vi "FPGA Main Default.vi"() -> ()   [LabVIEW 2021]
doc: "The myRIO v1.1 FPGA Shipping Personality. This personality contains support for:\n- 2 Analog Input Interrupt channel\n- 4 Digital Input Interrupt channel\n- 1 Timer\n- 1 Accelerometer\n- 1 Button\n- 4 LED\n- 10 Analog Input channels with 1 Sample\n- 6 Analog Output channels with 1 Sample\n- 40 Digital I/O channels with 1 Sample\n- 2 I2C channels\n- 4 Encoder channels\n- 6 PWM channels\n- 2 SPI channels"
uses:
  Sub VIs/Utilities/Start Boolean.ctl
  <vilib>/Platform/TimedLoop/XDataNode/timing_clust.ctl
  <vilib>/Platform/TimedLoop/XDataNode/nitl_modes.ctl
  <vilib>/Platform/TimedLoop/XDataNode/wakeup.ctl
  <vilib>/rvi/Emulation/niFpgaGetClockAttributes.vi
  <vilib>/rvi/Emulation/niFpgaSctlEmulationGetInTimedLoop.vi
  <vilib>/rvi/Emulation/niFpgaEmulationReportErrorSimple.vi
  <vilib>/rvi/eio/common/nirviEmuTemplateMethod_errors.vi
  <vilib>/rvi/Emulation/niFpgaCriticalErrorInLSC.vi
  <vilib>/rvi/Emulation/niFpgaProcessEmulError.vi
  <vilib>/rvi/Emulation/niFpgaEmulationIsFPGAContextNoSignature.vi
  <vilib>/rvi/errors/niFpgaSetErrorForExecOnDevCompSimple.vi
  <vilib>/rvi/eio/common/nirviEmuReportErrorAndStop.vi
  <vilib>/rvi/DataTransferAndStorage/Container/Common/niFpgaContainerGetUniqueNameForEmu.vi
  <vilib>/rvi/FIFO/Fifo_Resource/nirvififoEmulationSetSize.vi
  <vilib>/rvi/FIFO/Fifo_Resource/nirviFifoEmulationQueueMgr.vi
  <instcachedir>/0/nirviFifoEmulationQueueMgr_E5CAEC123FF24DC58D834DCA3CDAA9B5.lvgen/nirviFifoEmulationQueueMgr_E5CAEC123FF24DC58D834DCA3CDAA9B5_000.vi
  <vilib>/rvi/FIFO/Fifo_Resource/nirvififoEmulationDetermineInputValidOut.vi
  <vilib>/rvi/FIFO/Fifo_Resource/nirvififoEmulationCreateLock.vi
  <vilib>/rvi/FIFO/Fifo_Resource/nirvififoEmulationObtainLock.vi
  <vilib>/rvi/FIFO/Fifo_Resource/nirvififoEmulationReleaseLock.vi
  <vilib>/rvi/occurrence/nirviWaitOnOccurrenceBase.vi
  <vilib>/rvi/errors/nirviReportUnexpectedCaseInternalError.vi
  <vilib>/rvi/errors/nirviReportUnexpectedCaseInternalError (U32).vi
  <vilib>/Utility/error.llb/Clear Errors.vi
  <vilib>/rvi/DataTransferAndStorage/Container/Common/niFpgaContainerSetEmuInfo.vi
  <vilib>/eio/EIONode/EIONode.xnode
  <vilib>/rvi/DataTransferAndStorage/Container/XNode/niFpgaContainer.xnode
  <vilib>/rvi/FIFO/Fifo_Resource/nirvififoEmulationWrite.vi
  <vilib>/rvi/FIFO/Fifo_Resource/nirvififoEmulationRead.vi
  <vilib>/Platform/TimedLoop/XDataNode/XDataNode.xnode
  <vilib>/rvi/LocalResourceManager/LocalResourceManager.xnode
  <vilib>/Platform/TimedLoop/XDataNode/XDNodeRunTimeDep.lvlib
panel:
  in  "AO.A_0.VAL":u16
  in  "AO.A_1.VAL":u16
  in  "AO.B_0.VAL":u16
  in  "AO.B_1.VAL":u16
  out "AI.B_3.VAL":u16
  out "AI.B_2.VAL":u16
  out "AI.B_1.VAL":u16
  out "AI.B_0.VAL":u16
  out "AI.A_3.VAL":u16
  out "AI.A_2.VAL":u16
  out "AI.A_1.VAL":u16
  out "AI.A_0.VAL":u16
  out "DIO.B_7:0.IN":u8 format="%08b"
  in  "DIO.B_7:0.DIR":u8 format="%08b"
  in  "DIO.B_7:0.OUT":u8 format="%08b"
  in  "PWM.A_2.CS":u8=1
  in  "PWM.A_2.CNFG":u8=4
  out "PWM.A_2.CNTR":u16
  in  "PWM.A_2.MAX":u16=39999
  in  "PWM.A_2.CMP":u16=20000
  in  "PWM.A_1.CS":u8=1
  in  "PWM.A_1.CNFG":u8=4
  out "PWM.A_1.CNTR":u16
  in  "PWM.A_1.MAX":u16=39999
  in  "PWM.A_1.CMP":u16=20000
  in  "PWM.A_0.CS":u8=1
  in  "PWM.A_0.CNFG":u8=4
  out "PWM.A_0.CNTR":u16
  in  "PWM.A_0.CMP":u16=20000
  in  "PWM.A_0.MAX":u16=39999
  in  "SPI.A.DATO":u16
  out "SPI.A.DATI":u16
  in  "SPI.A.CNFG":u16=112
  in  "SPI.A.CNT":u16=19
  in  "SPI.B.CNT":u16=19
  in  "SPI.B.CNFG":u16=112 format="%0.0f"
  out "SPI.B.DATI":u16
  in  "SPI.B.DATO":u16
  in  "ENC.A.CNFG":u8 format="%08b"
  in  "ENC.B.CNFG":u8 format="%08b"
  out "ENC.A.CNTR":u32
  out "ENC.B.CNTR":u32
  out "ENC.A.STAT":u8 format="%08b"
  out "ENC.B.STAT":u8 format="%08b"
  in  "SPI.A.GO":T1
  out "SPI.A.STAT":u8 format="%08b"
  in  "SPI.B.GO":T1
  out "SPI.B.STAT":u8 format="%08b"
  out "I2C.B.STAT":u8 format="%08b"
  in  "I2C.B.CNTL":u8 format="%08b"
  out "I2C.A.STAT":u8 format="%08b"
  in  "I2C.A.CNTL":u8 format="%08b"
  in  "I2C.B.CNTR":u8=213
  in  "I2C.B.ADDR":u8 format="%08.0f"
  out "I2C.B.DATI":u8
  in  "I2C.B.DATO":u8
  in  "I2C.A.CNTR":u8=213
  in  "I2C.A.ADDR":u8 format="%08b"
  out "I2C.A.DATI":u8
  in  "I2C.A.DATO":u8
  in  "I2C.B.CNFG":u8=1 format="%08b"
  in  "I2C.A.CNFG":u8=1 format="%08b"
  in  "I2C.A.GO":T1
  in  "I2C.B.GO":T1
  out "SYS.AI.RDY":bool
  out "SYS.RDY":bool
  in  "PWM.B_2.CS":u8=1
  in  "PWM.B_2.CNFG":u8=4
  out "PWM.B_2.CNTR":u16
  in  "PWM.B_2.MAX":u16=39999
  in  "PWM.B_2.CMP":u16=20000
  in  "PWM.B_1.CS":u8=1
  in  "PWM.B_1.CNFG":u8=4
  out "PWM.B_1.CNTR":u16
  in  "PWM.B_1.MAX":u16=39999
  in  "PWM.B_1.CMP":u16=20000
  in  "PWM.B_0.CS":u8=1
  in  "PWM.B_0.CNFG":u8=4
  out "PWM.B_0.CNTR":u16
  in  "PWM.B_0.MAX":u16=39999
  in  "PWM.B_0.CMP":u16=20000
  out "DIO.A_7:0.IN":u8 format="%08b"
  in  "DIO.A_7:0.OUT":u8 format="%08b"
  in  "DIO.A_7:0.DIR":u8 format="%08b"
  out "DIO.C_7:0.IN":u8 format="%08b"
  in  "DIO.C_7:0.DIR":u8 format="%08b"
  in  "DIO.C_7:0.OUT":u8 format="%08b"
  out "AI.C_1.VAL":u16
  out "AI.C_0.VAL":u16
  in  "AO.C_0.VAL":u16
  in  "AO.C_1.VAL":u16
  in  "SYS.SELECTB":u8 format="%08b"
  in  "SYS.SELECTC":u8 format="%08b"
  in  "SYS.SELECTA":u8 format="%08b"
  in  "ENC.C_0.CNFG":u8 format="%08b"
  out "ENC.C_0.CNTR":u32
  out "ENC.C_0.STAT":u8 format="%08b"
  in  "ENC.C_1.CNFG":u8 format="%08b"
  out "ENC.C_1.CNTR":u32
  out "ENC.C_1.STAT":u8 format="%08b"
  in  "PWM.C_1.CS":u8=1
  in  "PWM.C_1.CNFG":u8=4
  out "PWM.C_1.CNTR":u16
  in  "PWM.C_1.CMP":u16=20000
  in  "PWM.C_1.MAX":u16=39999
  in  "PWM.C_0.CS":u8=1
  in  "PWM.C_0.CNFG":u8=4
  out "PWM.C_0.CNTR":u16
  in  "PWM.C_0.CMP":u16=20000
  in  "PWM.C_0.MAX":u16=39999
  out "DIO.A_15:8.IN":u8 format="%08b"
  in  "DIO.A_15:8.OUT":u8 format="%08b"
  in  "DIO.A_15:8.DIR":u8 format="%08b"
  out "DIO.B_15:8.IN":u8 format="%08b"
  in  "DIO.B_15:8.DIR":u8 format="%08b"
  in  "DIO.B_15:8.OUT":u8 format="%08b"
  out "AI.AudioIn_R.VAL":u16
  out "AI.AudioIn_L.VAL":u16
  in  "AO.AudioOut_R.VAL":u16
  in  "AO.AudioOut_L.VAL":u16
  in  "AO.SYS.GO":T1
  out "ACC.X.VAL":u16
  out "ACC.Y.VAL":u16
  out "SYS.ACC.RDY":bool
  out "ACC.Z.VAL":u16
  in  "DO.LED3:0":u8 format="%04b"
  out "DI.BTN":u8 format="%08b"
  out "AO.SYS.STAT":bool
  in  "IRQ.AI_A_3:0.CNFG":u8 format="%.0b"
  in  "IRQ.AI_A_0.THRESHOLD":u16
  in  "IRQ.AI_A_1.THRESHOLD":u16
  in  "IRQ.AI_A_0.NO":u8
  in  "IRQ.AI_A_1.NO":u8
  in  "IRQ.DIO_A_7:0.ENA":u8 format="%08b"
  in  "IRQ.DIO_A_7:0.RISE":u8 format="%08b"
  in  "IRQ.DIO_A_7:0.FALL":u8 format="%08b"
  in  "IRQ.DIO_A_0.NO":u8
  in  "IRQ.DIO_A_1.NO":u8
  in  "IRQ.DIO_A_2.NO":u8
  in  "IRQ.DIO_A_3.NO":u8
  in  "IRQ.DIO_A_3.CNT":u32
  in  "IRQ.DIO_A_2.CNT":u32
  in  "IRQ.DIO_A_1.CNT":u32
  in  "IRQ.DIO_A_0.CNT":u32
  in  "IRQ.AI_A_1.HYSTERESIS":u16=17
  in  "IRQ.TIMER.WRITE":u32
  in  "IRQ.TIMER.SETTIME":T1
  out "IRQ.TIMER.READ":u32
  in  "SPI.A.IRQ.NO":u8=15
  in  "SPI.B.IRQ.NO":u8=15
  in  "IRQ.AI_A_0.HYSTERESIS":u16=17
  in  "IRQ.DI_BTN.ENA":bool
  in  "IRQ.DI_BTN.RISE":bool
  in  "IRQ.DI_BTN.FALL":bool
  in  "IRQ.DI_BTN.CNT":u32
  in  "IRQ.DI_BTN.NO":u8
  # "System"
  # "Onboard Devices"
  # "Connector A"
  # "Connector B"
  # "Connector C"
  # "Audio Connector"
  # "Accelerometer"
  # "Analog Input"
  # "Analog Output"
  # "Digital I/O"
  # "PWM"
  # "SPI Master"
  # "Analog Input"
  # "Analog Output"
  # "Digital I/O"
  # "PWM"
  # "SPI Master"
  # "Analog Input"
  # "Analog Output"
  # "Digital I/O"
  # "Counters / PWM"
  # "Analog Input"
  # "Analog Output"
  # "IO Configuration"
  # "IO Configuration"
  # "IO Configuration"
  # "Encoders"
  # "Buttons & LEDs"
  # "Analog Interrupt"
  # "Digital Interrupt"
  # "Encoders"
  # "Encoders"
  # "Button Interrupt"
  # "I2C Master"
  # "I2C Master"
  # "Timer Interrupt"
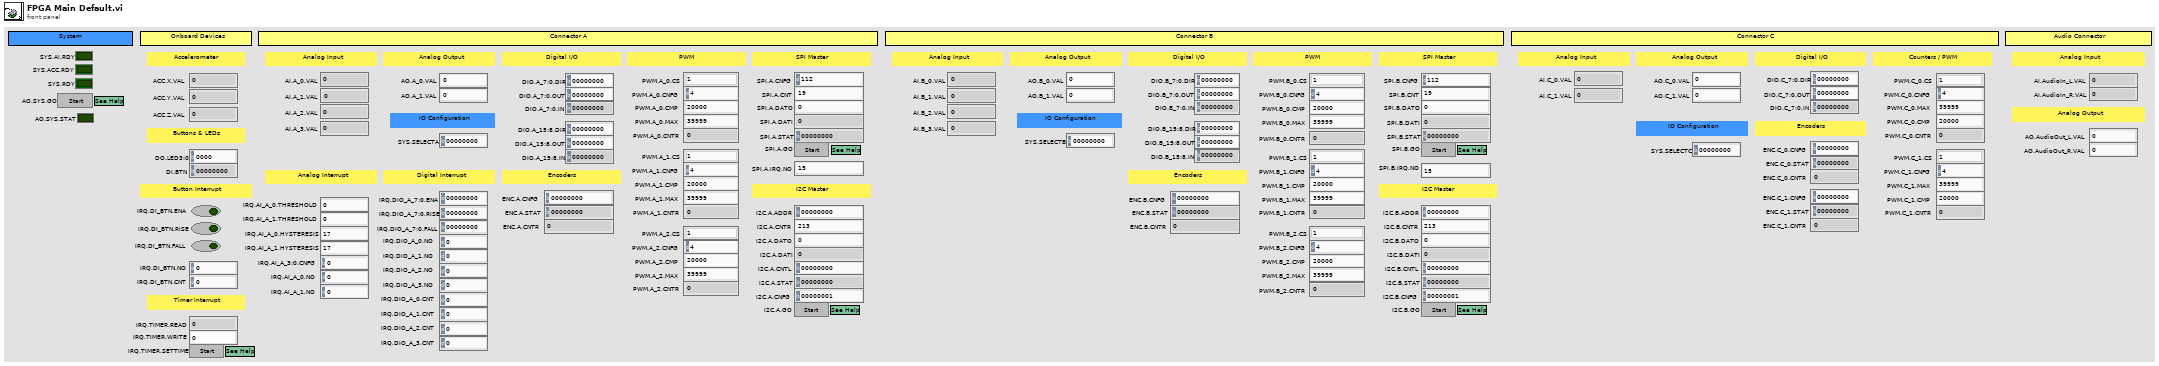
[diagram p1: front panel]
types:
  T1 = typedef "Start Boolean.ctl" = bool
  T2 = typedef "XDNodeRunTimeDep.lvlib/timing_clust.ctl" = cluster{"Expected End [f-1]":u64, "Actual End [f-1]":u64, "Finished Late? [f-1]":bool, "Expected End [i-1]":u64, "Actual End [i-1]":u64, "Finished Late? [i-1]":bool, "Expected Start [i]":u64, "Actual Start [i]":u64, "Expected Start [f]":u64, "Actual Start [f]":u64, "Source Name":string, "Structure Name":string, "Period":i64, "Deadline":i64, "Offset":i64, "Start":i64, "Priority":i32, "Timeout":i32, "Mode":T3, "Wakeup Reason":T4, "Error":errorcluster, "Source Type":string, "Secondary Source Type":string, "Global End Time":u64, "Global Start Time":u64, "Frame Duration":u64, "Iteration Duration":u64, "Assigned CPU":i32, "I/O Scan Engine Mode":u32}
  T3 = typedef "XDNodeRunTimeDep.lvlib/nitl_modes.ctl" = enum32{"No Change", "Process missed periods, maintain original phase", "Discard missed periods, maintain original phase", "Process missed periods, ignore original phase", "Discard missed periods, ignore original phase"}
  T4 = typedef "XDNodeRunTimeDep.lvlib/wakeup.ctl" = enum32{"Normal", "Aborted", "Asynchronous wakeup", "Timing source error", "Timed loop error", "Timeout"}
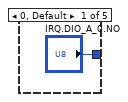
[diagram p9: hidden frame]
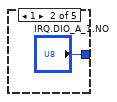
[diagram p10: hidden frame]
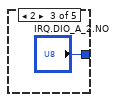
[diagram p11: hidden frame]
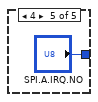
[diagram p12: hidden frame]
diagram:
  # "The Timed Loop does not allow writing the same FIFO outside the Timed Loop. Use another FIFO to push all interrupts from DIO in the Timed Loop to the IRQ Queue."
  # "The Timed Loop does not allow writing the same FIFO outside the Timed Loop. Use another FIFO to push all interrupts from Button in the Timed Loop to the IRQ Queue."
  # "The Timed Loop does not allow writing the same FIFO outside the Timed Loop. Use another FIFO to push all interrupts from DIO in the Timed Loop to the IRQ Queue."
  # "The accelerometer nodes take some time before the FPGA can first read the values. This is because it takes time to read from the accelerometer. An iteration of the While Loop will not complete until the accelerometer values have been read.\n\nAfter the completion of the first iteration of the While Loop, all indicators have valid values."
  # "The analog output nodes take some time before the FPGA write the values to the pins. The GO and STAT registers are used to handshake between the FPGA and host. When the host wants the values to be written, the host sets the GO register to TRUE. If the host reads the STAT register before setting the value of the GO register, it can wait for the value of the STAT register to invert. The value inversion tells the host that the output values have been written."
  # "The analog input nodes take some time before the FPGA can first read the values. This is because it takes time to set up the Analog-to-Digital converter (ADC) and convert the first reading. An iteration of the While Loop will not complete until all the analog input channels have been sampled.\n\nAfter the completion of the first iteration of the While Loop, all indicators have valid values."
  # "Note: On some hardware a \"ghosting effect\" may occur on any unconnected AI channels. For example, if channel AI0 is connected and channels AI1~AI7 are not connected the the value read at AI0 may be seen on indicators AI1~AI7. This is common for hardware that use a multiplexed (MUXed) Analog-to-Digital converter (ADC), because the input analog signal is used to charge a capacitor which does not discharge before the unconnected channel is read.\n\nYou can hide the \"ghosting effect\" by using an mask register. This register is used to decide when the indicator should be updated."
  # "The FPGA timer fires the interrupt request (IRQ) when TIMER.Read counts down to zero. If TIMER.Read is not zero, it counts down to one per microsecond."
  # "The only interface that sends interrupts to the RT side. Timer interrupts, analog input interrupts, digital input interrupts, and SPI interrupt share this interface.\n\nAll interrupts work in sequence. One interrupt waits until the previous interrupt request (IRQ) gets acknowledged on the RT side."
  # "NOTE: The SYS.RDY Boolean MUST exist and must become TRUE at some point. Otherwise, the myRIO VIs will not function correctly."
  # "There is some delay between the time when the FPGA code starts and the time when the analog inputs, accelerometer, and scaling values outputs are valid. If the host wants to ensure that there are valid values in theses registers it should wait for each subsystem to finish its initialization process. \n\nWhen all subsystems have finished initializinig, the SYS.RDY indicator turns true. The host can poll the SYS.RDY indicator to determine the status of the FPGA. Alternatively, the host can poll the individual SYS.xx.RDY indicators to determine the status of the individual subsystems.\n\nThis loop continues indefinitely, essentially making SYS.RDY a read-only register."
  n1 = while {
    stop <- FALSE stop-if-true
    # "Host Synchronization"
    n2 = local read "SYS.ACC.RDY"() -> (w13:bool)
    n3 = local read "SYS.AI.RDY"() -> (w15:bool)
    n4 = Compound Arithmetic op=AND(w15, w13) -> (→"SYS.RDY":bool)
  }
  n5 = while {
    stop <- FALSE stop-if-true
    # "Interrupt to RT"
    n6 = xnode ("FIFO Method Node")("Timeout"=-1) -> ("Element"=w18:u8)  [unwired: 1 in, 2 out]
    n7 = call <vilib>:"niFPGA Interrupt.vi"("Wait Until Cleared (F)"=TRUE, "IRQ Number (0)"=w18) -> ()  [unwired: 1 in]
  }
  n8 = while {
    stop <- FALSE stop-if-true
    # "Timer"
    n9 = local read "IRQ.TIMER.READ"() -> (w23:u32)
    n10 = Select(t="IRQ.TIMER.WRITE", s="IRQ.TIMER.SETTIME", f=w23) -> (s? t:f=w21:u32)
    n11 = case shown="Default" w21 {
      selector: w21 -> [w27 w30]
      tunnel: [w27 w28] -> w20
      frame 0 {
      }
      frame Default {
        n12 = Decrement(x=w30) -> (x-1=w29:u32)
        n13 = case shown="0" w29 {
          selector: w29 -> [w31 w34]
          tunnel: [w31 w34] -> w28
          frame Default {
          }
          frame 0 {
            w33 = u8 0  # Reserved for Timer IRQ
            n14 = xnode ("FIFO Method Node")("Element"=w33, "Timeout"=-1) -> ()  [unwired: 1 in, 2 out]
          }
        }
      }
    }
    "IRQ.TIMER.READ" <- w20
    n15 = call "Loop Timer"("Count(uSec)"=u8 1 ("Count(mSec)")) -> ()  [unwired: 1 out]
  }
  n16 = xnode "VI-Defined FIFO Configuration"() -> ("FIFO Out"=w3:refnum<k21>)
  n17 = while {
    tunnel: w3 -> [w36]
    i -> [w63]
    stop <- FALSE stop-if-true
    # "Analog Input"
    n18 = xnode "FPGA I/O Node"() -> ("ConnectorA/AI0"=w41:u16, "ConnectorA/AI1"=w40:u16, "ConnectorA/AI2"=→"AI.A_2.VAL":u16, "ConnectorA/AI3"=→"AI.A_3.VAL":u16, "ConnectorB/AI0"=→"AI.B_0.VAL":u16, "ConnectorB/AI1"=→"AI.B_1.VAL":u16, "ConnectorB/AI2"=→"AI.B_2.VAL":u16, "ConnectorB/AI3"=→"AI.B_3.VAL":u16, "ConnectorC/AI0"=w57:i16, "ConnectorC/AI1"=w56:i16, "AudioIn/Left"=w55:i16, "AudioIn/Right"=w54:i16)  [unwired: 12 in, 12 out]
    "AI.A_0.VAL" <- w41
    "AI.A_1.VAL" <- w40
    n19 = Greater Than 0?(x=w63) -> (x > 0?=→"SYS.AI.RDY":bool)
    n20 = Number To Boolean Array(number="IRQ.AI_A_3:0.CNFG") -> (Boolean array=w51:bool[])
    n21 = Index Array(array=w51) -> (element #1=w49:bool, element #2=w48:bool, element #3=w46:bool, element #4=w45:bool)  [unwired: 4 in]
    n22 = To Unsigned Word Integer(number=w57) -> (unsigned 16bit integer=→"AI.C_0.VAL":u16)
    n23 = To Unsigned Word Integer(number=w56) -> (unsigned 16bit integer=→"AI.C_1.VAL":u16)
    n24 = To Unsigned Word Integer(number=w55) -> (unsigned 16bit integer=→"AI.AudioIn_L.VAL":u16)
    n25 = To Unsigned Word Integer(number=w54) -> (unsigned 16bit integer=→"AI.AudioIn_R.VAL":u16)
    n26 = call "Check AI IRQ.vi"("Hysteresis"="IRQ.AI_A_1.HYSTERESIS", "FIFO In"=w36, "IRQ Number"="IRQ.AI_A_1.NO", "Threshold"="IRQ.AI_A_1.THRESHOLD", "Analog Value"=w40, "Rising Edge?"=w45, "Enable Interrupt?"=w46) -> ()  [unwired: 5 in]
    n27 = call "Check AI IRQ.vi"("Hysteresis"="IRQ.AI_A_0.HYSTERESIS", "FIFO In"=w36, "IRQ Number"="IRQ.AI_A_0.NO", "Threshold"="IRQ.AI_A_0.THRESHOLD", "Analog Value"=w41, "Rising Edge?"=w48, "Enable Interrupt?"=w49) -> ()  [unwired: 5 in]
  }
  n28 = while {
    stop <- FALSE stop-if-true
    # "Analog Output"
    n29 = feedback #1(FALSE) -> (w69:bool)
    n30 = case shown="True" "AO.SYS.GO" {
      tunnel: "AO.C_0.VAL" -> [_ w91]
      tunnel: "AO.C_1.VAL" -> [_ w90]
      tunnel: "AO.A_0.VAL" -> [_ w95]
      tunnel: "AO.A_1.VAL" -> [_ w94]
      tunnel: "AO.B_0.VAL" -> [_ w93]
      tunnel: "AO.B_1.VAL" -> [_ w92]
      tunnel: "AO.AudioOut_L.VAL" -> [_ w87]
      tunnel: "AO.AudioOut_R.VAL" -> [_ w86]
      tunnel: w69 -> [w80 w83]
      tunnel: [w80 w81] -> w67
      frame False {
      }
      frame True {
        n31 = To Word Integer(number=w91) -> (16bit integer=w89:i16)
        n32 = To Word Integer(number=w90) -> (16bit integer=w88:i16)
        n33 = To Word Integer(number=w87) -> (16bit integer=w85:i16)
        n34 = To Word Integer(number=w86) -> (16bit integer=w84:i16)
        n35 = flat-sequence {
          tunnel: w95 -> [w104]
          tunnel: w94 -> [w103]
          tunnel: w93 -> [w102]
          tunnel: w92 -> [w101]
          tunnel: w89 -> [w100]
          tunnel: w88 -> [w99]
          tunnel: w85 -> [w98]
          tunnel: w84 -> [w97]
          tunnel: w83 -> [w96]
          tunnel: [w96] -> w82
          tunnel: w82 -> [w106]
          tunnel: [w105] -> w81
          frame #0 {
            n36 = xnode "FPGA I/O Node"("ConnectorA/AO0"=w104, "ConnectorA/AO1"=w103, "ConnectorB/AO0"=w102, "ConnectorB/AO1"=w101, "ConnectorC/AO0"=w100, "ConnectorC/AO1"=w99, "AudioOut/Left"=w98, "AudioOut/Right"=w97) -> ()  [unwired: 8 in, 8 out]
          }
          frame #1 {
            n37 = Not(x=w106) -> (.not. x?=w105:bool)
          }
        }
      }
    }
    "AO.SYS.STAT" <- w67
    n38 = feedback-in #1(w67) -> ()
  }
  n39 = while {
    i -> [w111]
    stop <- FALSE stop-if-true
    # "Onboard Accelerometer"
    n40 = xnode "FPGA I/O Node"() -> ("AccelerationX"=w114:i16, "AccelerationY"=w113:i16, "AccelerationZ"=w112:i16)  [unwired: 3 in, 3 out]
    n41 = Greater Than 0?(x=w111) -> (x > 0?=→"SYS.ACC.RDY":bool)
    n42 = To Unsigned Word Integer(number=w114) -> (unsigned 16bit integer=→"ACC.X.VAL":u16)
    n43 = To Unsigned Word Integer(number=w113) -> (unsigned 16bit integer=→"ACC.Y.VAL":u16)
    n44 = To Unsigned Word Integer(number=w112) -> (unsigned 16bit integer=→"ACC.Z.VAL":u16)
  }
  n45 = xnode "VI-Defined FIFO Configuration"() -> ("FIFO Out"=w2:refnum<k21>)
  n46 = node-c288() -> (w5:T2)  [unwired: 1 in]
  n47 = timed-loop {
    timing: w5 -> [_]
    timing-out: [_] -> w4
    tunnel: w2 -> [w118]
    stop <- _ stop-if-true
    # "Onboard DIO"
    n48 = xnode "FPGA I/O Node"() -> ("Button0"=w122:bool)  [unwired: 1 in, 1 out]
    n49 = Number To Boolean Array(number="DO.LED3:0") -> (Boolean array=w127:bool[])
    n50 = Build Array(w122) -> (w130:bool[])
    n51 = Index Array(array=w127) -> (element #1=w126:bool, element #2=w125:bool, element #3=w124:bool, element #4=w123:bool)  [unwired: 4 in]
    n52 = call "DIO IRQ 1-bit.vi"("IRQ.NO"="IRQ.DI_BTN.NO", "IRQ.CNT"="IRQ.DI_BTN.CNT", "FIFO in"=w118, "IRQ.FALL"="IRQ.DI_BTN.FALL", "IRQ.RISE"="IRQ.DI_BTN.RISE", "IRQ.ENA"="IRQ.DI_BTN.ENA", "DIO"=w122) -> ()  [unwired: 5 in]
    n53 = Boolean Array To Number(Boolean array=w130) -> (number=→"DI.BTN":u8)
    n54 = xnode "FPGA I/O Node"("LED0"=w126, "LED1"=w125, "LED2"=w124, "LED3"=w123) -> ()  [unwired: 4 in, 4 out]
  }
  n55 = while {
    stop <- FALSE stop-if-true
    # "Button SCTL Interrupt Buffer"
    n56 = feedback #2(u8 0 ("Element")) -> (w135:u8)
    n57 = feedback #3(FALSE ("Timed Out?")) -> (w139:bool)
    n58 = case shown="False" w139 {
      tunnel: [w141 w143] -> w136
      tunnel: w135 -> [_ w143]
      frame False {
        n59 = xnode ("FIFO Method Node")("Timeout"=-1) -> ("Element"=w141:u8)  [unwired: 1 in, 2 out]
      }
      frame True {
      }
    }
    n60 = feedback-in #2(w136) -> ()
    n61 = xnode ("FIFO Method Node")("Element"=w136, "Timeout"=0) -> ("Timed Out?"=w137:bool)  [unwired: 1 in, 1 out]
    n62 = feedback-in #3(w137) -> ()
  }
  n63 = node-c288(w4) -> ()
  n64 = node-c288() -> (w9:T2)  [unwired: 1 in]
  n65 = xnode "VI-Defined FIFO Configuration"() -> ()  [unwired: 1 out]
  n66 = while {
    stop <- FALSE stop-if-true
    # "Connector A SCTL Interrupt Buffer"
    n67 = feedback #4(u8 0 ("Element")) -> (w146:u8)
    n68 = feedback #5(FALSE ("Timed Out?")) -> (w150:bool)
    n69 = case shown="False" w150 {
      tunnel: [w152 w154] -> w147
      tunnel: w146 -> [_ w154]
      frame False {
        n70 = xnode ("FIFO Method Node")("Timeout"=-1) -> ("Element"=w152:u8)  [unwired: 1 in, 2 out]
      }
      frame True {
      }
    }
    n71 = feedback-in #4(w147) -> ()
    n72 = xnode ("FIFO Method Node")("Element"=w147, "Timeout"=0) -> ("Timed Out?"=w148:bool)  [unwired: 1 in, 1 out]
    n73 = feedback-in #5(w148) -> ()
  }
  n74 = timed-loop {
    timing: w9 -> [_]
    timing-out: [_] -> w8
    stop <- _ stop-if-true
    w155 = u16 5 ("Debounce Ticks")
    w156 = u8 0
    # "Trigger the interrupt at next \ntick if timeout"
    # "DIO / Encoder"
    # "DIO / I2C Master"
    # "DIO / PWM"
    # "DIO"
    # "DIO"
    # "DIO/ SPI Master"
    # "Connector A DIO"
    n75 = call "Split HDC Bank1 DIO.vi"("IN 7:0"="DIO.A_7:0.OUT") -> ("OUT 3:0"=w291:fxp<+,4,4>, "OUT 4"=w210:bool, "OUT 7:5"=w288:fxp<+,3,3>)
    n76 = call "Split HDC Bank1 DIO.vi"("IN 7:0"="DIO.A_7:0.DIR") -> ("OUT 3:0"=w290:fxp<+,4,4>, "OUT 4"=w289:bool, "OUT 7:5"=w287:fxp<+,3,3>)
    n77 = call "Split HDC Function Select.vi"("IN 7:0"="SYS.SELECTA") -> ("OUT 1:0"=w230:fxp<+,2,2>, "OUT 7"=w225:bool, "OUT 2"=w229:bool, "OUT 3"=w228:bool, "OUT 4"=w227:bool, "OUT 5"=w226:bool)
    n78 = call "DIO 4-bit.vi"("DIO0 Refnum"=refnum<k21> "ConnectorA/DIO0", "DIO1 Refnum"=refnum<k21> "ConnectorA/DIO1", "DIO2 Refnum"=refnum<k21> "ConnectorA/DIO2", "DIR 3:0"=w290, "OUT 3:0"=w291, "DIO3 Refnum"=refnum<k21> "ConnectorA/DIO3") -> ("IN 3:0"=w178:fxp<+,4,4>)  [unwired: 5 in]
    n79 = call "DIO 1-bit.vi"("DIR"=w289, "OUT"=w210, "DIO Refnum"=refnum<k21> "ConnectorA/DIO4") -> ("IN"=w177:bool)  [unwired: 8 in]
    n80 = call "DIO_SPI.vi"("DIO.2:0.OUT"=w288, "DIO.2:0.DIR"=w287, "SPI.CNT"="SPI.A.CNT", "SPI.CNFG"="SPI.A.CNFG", "SPI.DATO"="SPI.A.DATO", "SPI.GO"="SPI.A.GO", "DIO.2/SPI.MOSI Refnum"=refnum<k21> "ConnectorA/DIO7" ("DIO.2/SPI.SCLK"), "SELECT.1:0"=w230, "DIO.1/SPI.MISO Refnum"=refnum<k21> "ConnectorA/DIO6" ("DIO.1/SPI.MOSI"), "DIO.0/SPI.SCLK Refnum"=refnum<k21> "ConnectorA/DIO5" ("DIO.0/SPI.MISO")) -> ("DIO.2:0.IN"=w263:fxp<+,3,3>, "SPI.DATI"=→"SPI.A.DATI":u16, "SPI.STAT"=w163:u8)  [unwired: 7 in]
    "SPI.A.STAT" <- w163
    n81 = Number To Boolean Array(number=w163) -> (Boolean array=w165:bool[])
    n82 = Index Array(array=w165) -> (element=w164:bool)  [unwired: 1 in]
    n83 = call "Falling Edge Trigger.vi"("Signal"=w164) -> ("Trigger?"=w162:bool)
    n84 = call "Join HDC Bank1 DIO.vi"("IN 7:5"=w263, "IN 4"=w177, "IN 3:0"=w178) -> ("OUT 7:0"=→"DIO.A_7:0.IN":u8)
    n85 = Number To Boolean Array(number=w178) -> (Boolean array=w203:bool[])
    n86 = Number To Boolean Array(number="IRQ.DIO_A_7:0.ENA") -> (Boolean array=w209:bool[])
    n87 = Number To Boolean Array(number="IRQ.DIO_A_7:0.RISE") -> (Boolean array=w208:bool[])
    n88 = Number To Boolean Array(number="IRQ.DIO_A_7:0.FALL") -> (Boolean array=w207:bool[])
    n89 = call "Split HDC Bank2 DIO.vi"("IN 7:0"="DIO.A_15:8.OUT") -> ("OUT 5"=w212:bool, "OUT 7:6"=w234:fxp<+,2,2>, "OUT 4:3"=w214:fxp<+,2,2>, "OUT 2"=w216:bool, "OUT 0"=w220:bool, "OUT 1"=w219:bool)  [unwired: 2 in]
    n90 = call "Split HDC Bank2 DIO.vi"("IN 7:0"="DIO.A_15:8.DIR") -> ("OUT 5"=w211:bool, "OUT 7:6"=w233:fxp<+,2,2>, "OUT 4:3"=w213:fxp<+,2,2>, "OUT 2"=w215:bool, "OUT 0"=w218:bool, "OUT 1"=w217:bool)  [unwired: 2 in]
    n91 = Index Array(array=w203) -> (element #1=w184:bool, element #2=w199:bool, element #3=w198:bool, element #4=w197:bool)  [unwired: 4 in]
    n92 = Index Array(array=w209) -> (element #1=w202:bool, element #2=w196:bool, element #3=w195:bool, element #4=w194:bool)  [unwired: 4 in]
    n93 = Index Array(array=w208) -> (element #1=w201:bool, element #2=w193:bool, element #3=w192:bool, element #4=w191:bool)  [unwired: 4 in]
    n94 = Index Array(array=w207) -> (element #1=w200:bool, element #2=w190:bool, element #3=w189:bool, element #4=w188:bool)  [unwired: 4 in]
    n95 = call "Check DI IRQ.vi"("Debounce Ticks"=w155, "Count"="IRQ.DIO_A_0.CNT", "On Falling Edge?"=w200, "On Rising Edge?"=w201, "Enable Interrupt?"=w202, "Digital In"=w184) -> ("Trigger?"=w175:bool)  [unwired: 5 in]
    n96 = call "Check DI IRQ.vi"("Debounce Ticks"=w155, "Count"="IRQ.DIO_A_1.CNT", "On Falling Edge?"=w190, "On Rising Edge?"=w193, "Enable Interrupt?"=w196, "Digital In"=w199) -> ("Trigger?"=w174:bool)  [unwired: 5 in]
    n97 = call "Check DI IRQ.vi"("Debounce Ticks"=w155, "Count"="IRQ.DIO_A_2.CNT", "On Falling Edge?"=w189, "On Rising Edge?"=w192, "Enable Interrupt?"=w195, "Digital In"=w198) -> ("Trigger?"=w173:bool)  [unwired: 5 in]
    n98 = call "DIO_PWM.vi"("DIO.OUT"=w220, "DIO.DIR"=w218, "PWM.CS"="PWM.A_0.CS", "PWM.CNFG"="PWM.A_0.CNFG", "PWM.CMP"="PWM.A_0.CMP", "PWM.MAX"="PWM.A_0.MAX", "DIO/PWM"=refnum<k21> "ConnectorA/DIO8", "SELECT"=w229) -> ("DIO.IN"=w224:bool, "PWM.CNTR"=→"PWM.A_0.CNTR":u16)  [unwired: 10 in]
    n99 = call "DIO_PWM.vi"("DIO.OUT"=w219, "DIO.DIR"=w217, "PWM.CS"="PWM.A_1.CS", "PWM.CNFG"="PWM.A_1.CNFG", "PWM.CMP"="PWM.A_1.CMP", "PWM.MAX"="PWM.A_1.MAX", "DIO/PWM"=refnum<k21> "ConnectorA/DIO9", "SELECT"=w228) -> ("DIO.IN"=w223:bool, "PWM.CNTR"=→"PWM.A_1.CNTR":u16)  [unwired: 10 in]
    n100 = call "DIO_PWM.vi"("DIO.OUT"=w216, "DIO.DIR"=w215, "PWM.CS"="PWM.A_2.CS", "PWM.CNFG"="PWM.A_2.CNFG", "PWM.CMP"="PWM.A_2.CMP", "PWM.MAX"="PWM.A_2.MAX", "DIO/PWM"=refnum<k21> "ConnectorA/DIO10", "SELECT"=w227) -> ("DIO.IN"=w222:bool, "PWM.CNTR"=→"PWM.A_2.CNTR":u16)  [unwired: 10 in]
    n101 = call "Check DI IRQ.vi"("Debounce Ticks"=w155, "Count"="IRQ.DIO_A_3.CNT", "On Falling Edge?"=w188, "On Rising Edge?"=w191, "Enable Interrupt?"=w194, "Digital In"=w197) -> ("Trigger?"=w172:bool)  [unwired: 5 in]
    n102 = feedback #6(w156) -> (w158:u8)
    n103 = Less?(x=w158, y=4 ("x")) -> (x < y?=w160:bool)
    n104 = Increment(x=w158) -> (x+1=w159:u8)
    n105 = Select(t=w159, s=w160, f=w156) -> (s? t:f=w157:u8)
    n106 = feedback-in #6(w157) -> ()
    n107 = case shown="3" w158 {
      tunnel: ["IRQ.DIO_A_0.NO" "IRQ.DIO_A_1.NO" "IRQ.DIO_A_2.NO" "IRQ.DIO_A_3.NO" "SPI.A.IRQ.NO"] -> w187
      frame 0, Default {
      }
      frame 1 {
      }
      frame 2 {
      }
      frame 3 {
      }
      frame 4 {
      }
    }
    n108 = Build Array(w175, w174, w173, w172, w162) -> (w170:bool[])
    n109 = call "DIO_Encoder.vi"("DIO.1:0.OUT"=w214, "DIO.1:0.DIR"=w213, "QE.CNFG"="ENC.A.CNFG", "DIO.1/QE.B"=refnum<k21> "ConnectorA/DIO12", "SELECT"=w226, "DIO.0/QE.A"=refnum<k21> "ConnectorA/DIO11") -> ("DIO.1:0.IN"=w221:fxp<+,2,2>, "QE.CNTR"=→"ENC.A.CNTR":u32, "QE.STAT"=→"ENC.A.STAT":u8)  [unwired: 11 in]
    n110 = call "DIO 1-bit.vi"("DIR"=w211, "OUT"=w212, "DIO Refnum"=refnum<k21> "ConnectorA/DIO13") -> ("IN"=w176:bool)  [unwired: 8 in]
    n111 = call "DIO_I2C.vi"("DIO.1:0.OUT"=w234, "DIO.1:0.DIR"=w233, "I2C.CNFG"="I2C.A.CNFG", "I2C.CNTL"="I2C.A.CNTL", "I2C.ADDR"="I2C.A.ADDR", "I2C.DATO"="I2C.A.DATO", "DIO.1/I2C.SDA"=refnum<k21> "ConnectorA/DIO15" ("DIO.1/I2C.SCL"), "I2C.CNTR"="I2C.A.CNTR", "DIO.0/I2C.SCL"=refnum<k21> "ConnectorA/DIO14" ("DIO.0/I2C.SDA"), "Execute?"="I2C.A.GO", "SELECT"=w225) -> ("DIO.1:0.IN"=w232:fxp<+,2,2>, "I2C.DATI"=→"I2C.A.DATI":u8, "I2C.STAT"=→"I2C.A.STAT":u8)  [unwired: 6 in]
    n112 = feedback #7(bool[] [FALSE, FALSE, FALSE, FALSE, FALSE] ("initialized array")) -> (w166:bool[])
    n113 = Or(x=w170, y=w166) -> (x .or. y?=w171:bool[])
    n114 = Index Array(array=w171, index=w158) -> (element=w169:bool)
    n115 = case shown="True" w169 {
      selector: w169 -> [w292 _]
      tunnel: [w292 w293] -> w168
      tunnel: w187 -> [_ w294]
      frame False {
      }
      frame True {
        n116 = xnode ("FIFO Method Node")("Element"=w294, "Timeout"=0) -> ("Timed Out?"=w293:bool)  [unwired: 1 in, 1 out]
      }
    }
    n117 = Replace Array Subset(array=w171, new element=w168, index=w158) -> (w167:bool[])
    n118 = feedback-in #7(w167) -> ()
    n119 = call "Join HDC Bank2 DIO.vi"("IN 7:6"=w232, "IN 5"=w176, "IN 4:3"=w221, "IN 0"=w224, "IN 2"=w222, "IN 1"=w223) -> ("OUT 7:0"=→"DIO.A_15:8.IN":u8)  [unwired: 4 in]
  }
  n120 = node-c288(w8) -> ()
  n121 = xnode "VI-Defined FIFO Configuration"() -> ("FIFO Out"=w1:refnum<k21>)
  n122 = node-c288() -> (w7:T2)  [unwired: 1 in]
  n123 = timed-loop {
    timing: w7 -> [_]
    timing-out: [_] -> w6
    tunnel: w1 -> [w303]
    stop <- _ stop-if-true
    # "DIO / Encoder"
    # "DIO / I2C Master"
    # "DIO / PWM"
    # "DIO"
    # "DIO"
    # "DIO/ SPI Master"
    # "Connector B DIO"
    n124 = call "Split HDC Bank1 DIO.vi"("IN 7:0"="DIO.B_7:0.OUT") -> ("OUT 3:0"=w392:fxp<+,4,4>, "OUT 4"=w390:bool, "OUT 7:5"=w388:fxp<+,3,3>)
    n125 = call "Split HDC Bank1 DIO.vi"("IN 7:0"="DIO.B_7:0.DIR") -> ("OUT 3:0"=w391:fxp<+,4,4>, "OUT 4"=w389:bool, "OUT 7:5"=w387:fxp<+,3,3>)
    n126 = call "Split HDC Function Select.vi"("IN 7:0"="SYS.SELECTB") -> ("OUT 1:0"=w364:fxp<+,2,2>, "OUT 7"=w359:bool, "OUT 2"=w363:bool, "OUT 3"=w362:bool, "OUT 4"=w361:bool, "OUT 5"=w360:bool)
    n127 = call "DIO 4-bit.vi"("DIO0 Refnum"=refnum<k21> "ConnectorB/DIO0", "DIO1 Refnum"=refnum<k21> "ConnectorB/DIO1", "DIO2 Refnum"=refnum<k21> "ConnectorB/DIO2", "DIR 3:0"=w391, "OUT 3:0"=w392, "DIO3 Refnum"=refnum<k21> "ConnectorB/DIO3") -> ("IN 3:0"=w370:fxp<+,4,4>)  [unwired: 5 in]
    n128 = call "DIO 1-bit.vi"("DIR"=w389, "OUT"=w390, "DIO Refnum"=refnum<k21> "ConnectorB/DIO4") -> ("IN"=w369:bool)  [unwired: 8 in]
    n129 = call "DIO_SPI.vi"("DIO.2:0.OUT"=w388, "DIO.2:0.DIR"=w387, "SPI.CNT"="SPI.B.CNT", "SPI.CNFG"="SPI.B.CNFG", "SPI.DATO"="SPI.B.DATO", "SPI.GO"="SPI.B.GO", "DIO.2/SPI.MOSI Refnum"=refnum<k21> "ConnectorB/DIO7" ("DIO.2/SPI.SCLK"), "SELECT.1:0"=w364, "DIO.1/SPI.MISO Refnum"=refnum<k21> "ConnectorB/DIO6" ("DIO.1/SPI.MOSI"), "DIO.0/SPI.SCLK Refnum"=refnum<k21> "ConnectorB/DIO5" ("DIO.0/SPI.MISO")) -> ("DIO.2:0.IN"=w368:fxp<+,3,3>, "SPI.DATI"=→"SPI.B.DATI":u16, "SPI.STAT"=w304:u8)  [unwired: 7 in]
    "SPI.B.STAT" <- w304
    n130 = call "SPI IRQ.vi"("SPI.A.IRQ.NO"="SPI.B.IRQ.NO", "SPI.STAT"=w304, "FIFO In"=w303) -> ()  [unwired: 9 in]
    n131 = call "Join HDC Bank1 DIO.vi"("IN 7:5"=w368, "IN 4"=w369, "IN 3:0"=w370) -> ("OUT 7:0"=→"DIO.B_7:0.IN":u8)
    n132 = call "Split HDC Bank2 DIO.vi"("IN 7:0"="DIO.B_15:8.OUT") -> ("OUT 5"=w316:bool, "OUT 7:6"=w367:fxp<+,2,2>, "OUT 4:3"=w317:fxp<+,2,2>, "OUT 2"=w318:bool, "OUT 0"=w320:bool, "OUT 1"=w319:bool)  [unwired: 2 in]
    n133 = call "Split HDC Bank2 DIO.vi"("IN 7:0"="DIO.B_15:8.DIR") -> ("OUT 5"=w311:bool, "OUT 7:6"=w366:fxp<+,2,2>, "OUT 4:3"=w312:fxp<+,2,2>, "OUT 2"=w313:bool, "OUT 0"=w315:bool, "OUT 1"=w314:bool)  [unwired: 2 in]
    n134 = call "DIO_PWM.vi"("DIO.OUT"=w320, "DIO.DIR"=w315, "PWM.CS"="PWM.B_0.CS", "PWM.CNFG"="PWM.B_0.CNFG", "PWM.CMP"="PWM.B_0.CMP", "PWM.MAX"="PWM.B_0.MAX", "DIO/PWM"=refnum<k21> "ConnectorB/DIO8", "SELECT"=w363) -> ("DIO.IN"=w310:bool, "PWM.CNTR"=→"PWM.B_0.CNTR":u16)  [unwired: 10 in]
    n135 = call "DIO_PWM.vi"("DIO.OUT"=w319, "DIO.DIR"=w314, "PWM.CS"="PWM.B_1.CS", "PWM.CNFG"="PWM.B_1.CNFG", "PWM.CMP"="PWM.B_1.CMP", "PWM.MAX"="PWM.B_1.MAX", "DIO/PWM"=refnum<k21> "ConnectorB/DIO9", "SELECT"=w362) -> ("DIO.IN"=w309:bool, "PWM.CNTR"=→"PWM.B_1.CNTR":u16)  [unwired: 10 in]
    n136 = call "DIO_PWM.vi"("DIO.OUT"=w318, "DIO.DIR"=w313, "PWM.CS"="PWM.B_2.CS", "PWM.CNFG"="PWM.B_2.CNFG", "PWM.CMP"="PWM.B_2.CMP", "PWM.MAX"="PWM.B_2.MAX", "DIO/PWM"=refnum<k21> "ConnectorB/DIO10", "SELECT"=w361) -> ("DIO.IN"=w308:bool, "PWM.CNTR"=→"PWM.B_2.CNTR":u16)  [unwired: 10 in]
    n137 = call "DIO_Encoder.vi"("DIO.1:0.OUT"=w317, "DIO.1:0.DIR"=w312, "QE.CNFG"="ENC.B.CNFG", "DIO.1/QE.B"=refnum<k21> "ConnectorB/DIO12", "SELECT"=w360, "DIO.0/QE.A"=refnum<k21> "ConnectorB/DIO11") -> ("DIO.1:0.IN"=w307:fxp<+,2,2>, "QE.CNTR"=→"ENC.B.CNTR":u32, "QE.STAT"=→"ENC.B.STAT":u8)  [unwired: 11 in]
    n138 = call "DIO 1-bit.vi"("DIR"=w311, "OUT"=w316, "DIO Refnum"=refnum<k21> "ConnectorB/DIO13") -> ("IN"=w306:bool)  [unwired: 8 in]
    n139 = call "DIO_I2C.vi"("DIO.1:0.OUT"=w367, "DIO.1:0.DIR"=w366, "I2C.CNFG"="I2C.B.CNFG", "I2C.CNTL"="I2C.B.CNTL", "I2C.ADDR"="I2C.B.ADDR", "I2C.DATO"="I2C.B.DATO", "DIO.1/I2C.SDA"=refnum<k21> "ConnectorB/DIO15" ("DIO.1/I2C.SCL"), "I2C.CNTR"="I2C.B.CNTR", "DIO.0/I2C.SCL"=refnum<k21> "ConnectorB/DIO14" ("DIO.0/I2C.SDA"), "Execute?"="I2C.B.GO", "SELECT"=w359) -> ("DIO.1:0.IN"=w365:fxp<+,2,2>, "I2C.DATI"=→"I2C.B.DATI":u8, "I2C.STAT"=→"I2C.B.STAT":u8)  [unwired: 6 in]
    n140 = call "Join HDC Bank2 DIO.vi"("IN 7:6"=w365, "IN 5"=w306, "IN 4:3"=w307, "IN 0"=w310, "IN 2"=w308, "IN 1"=w309) -> ("OUT 7:0"=→"DIO.B_15:8.IN":u8)  [unwired: 4 in]
  }
  n141 = while {
    stop <- FALSE stop-if-true
    # "Connector B SCTL Interrupt Buffer"
    n142 = feedback #8(u8 0 ("Element")) -> (w397:u8)
    n143 = feedback #9(FALSE ("Timed Out?")) -> (w401:bool)
    n144 = case shown="False" w401 {
      tunnel: [w403 w405] -> w398
      tunnel: w397 -> [_ w405]
      frame False {
        n145 = xnode ("FIFO Method Node")("Timeout"=-1) -> ("Element"=w403:u8)  [unwired: 1 in, 2 out]
      }
      frame True {
      }
    }
    n146 = feedback-in #8(w398) -> ()
    n147 = xnode ("FIFO Method Node")("Element"=w398, "Timeout"=0) -> ("Timed Out?"=w399:bool)  [unwired: 1 in, 1 out]
    n148 = feedback-in #9(w399) -> ()
  }
  n149 = node-c288(w6) -> ()
  n150 = node-c288() -> (w11:T2)  [unwired: 1 in]
  n151 = timed-loop {
    timing: w11 -> [_]
    timing-out: [_] -> w10
    stop <- _ stop-if-true
    # "Connector C  DIO"
    n152 = call "Split myDAQ DIO.vi"("IN 7:0"="DIO.C_7:0.OUT") -> ("OUT 2, OUT0"=w424:fxp<+,2,2>, "OUT 1"=w423:bool, "OUT 3"=w422:bool, "OUT 7"=w419:bool, "OUT 6, OUT 4"=w421:fxp<+,2,2>, "OUT 5"=w420:bool)  [unwired: 4 in]
    n153 = call "Split myDAQ DIO.vi"("IN 7:0"="DIO.C_7:0.DIR") -> ("OUT 2, OUT0"=w418:fxp<+,2,2>, "OUT 1"=w417:bool, "OUT 3"=w416:bool, "OUT 7"=w413:bool, "OUT 6, OUT 4"=w415:fxp<+,2,2>, "OUT 5"=w414:bool)  [unwired: 4 in]
    n154 = call "Split myDAQ Function Select.vi"("IN 7:0"="SYS.SELECTC") -> ("OUT 0"=w430:bool, "OUT 1"=w429:bool, "OUT 2"=w428:bool, "OUT 3"=w427:bool)  [unwired: 2 in]
    n155 = call "DIO_Encoder.vi"("DIO.1:0.OUT"=w424, "DIO.1:0.DIR"=w418, "QE.CNFG"="ENC.C_0.CNFG", "DIO.1/QE.B"=refnum<k21> "ConnectorC/DIO2", "SELECT"=w430, "DIO.0/QE.A"=refnum<k21> "ConnectorC/DIO0") -> ("DIO.1:0.IN"=w411:fxp<+,2,2>, "QE.CNTR"=→"ENC.C_0.CNTR":u32, "QE.STAT"=→"ENC.C_0.STAT":u8)  [unwired: 11 in]
    n156 = call "DIO 1-bit.vi"("DIR"=w417, "OUT"=w423, "DIO Refnum"=refnum<k21> "ConnectorC/DIO1") -> ("IN"=w410:bool)  [unwired: 8 in]
    n157 = call "DIO_PWM.vi"("DIO.OUT"=w422, "DIO.DIR"=w416, "PWM.CS"="PWM.C_0.CS", "PWM.CNFG"="PWM.C_0.CNFG", "PWM.CMP"="PWM.C_0.CMP", "PWM.MAX"="PWM.C_0.MAX", "DIO/PWM"=refnum<k21> "ConnectorC/DIO3", "SELECT"=w429) -> ("DIO.IN"=w409:bool, "PWM.CNTR"=→"PWM.C_0.CNTR":u16)  [unwired: 10 in]
    n158 = call "DIO_Encoder.vi"("DIO.1:0.OUT"=w421, "DIO.1:0.DIR"=w415, "QE.CNFG"="ENC.C_1.CNFG", "DIO.1/QE.B"=refnum<k21> "ConnectorC/DIO6", "SELECT"=w428, "DIO.0/QE.A"=refnum<k21> "ConnectorC/DIO4") -> ("DIO.1:0.IN"=w408:fxp<+,2,2>, "QE.CNTR"=→"ENC.C_1.CNTR":u32, "QE.STAT"=→"ENC.C_1.STAT":u8)  [unwired: 11 in]
    n159 = call "DIO 1-bit.vi"("DIR"=w414, "OUT"=w420, "DIO Refnum"=refnum<k21> "ConnectorC/DIO5") -> ("IN"=w407:bool)  [unwired: 8 in]
    n160 = call "DIO_PWM.vi"("DIO.OUT"=w419, "DIO.DIR"=w413, "PWM.CS"="PWM.C_1.CS", "PWM.CNFG"="PWM.C_1.CNFG", "PWM.CMP"="PWM.C_1.CMP", "PWM.MAX"="PWM.C_1.MAX", "DIO/PWM"=refnum<k21> "ConnectorC/DIO7", "SELECT"=w427) -> ("DIO.IN"=w406:bool, "PWM.CNTR"=→"PWM.C_1.CNTR":u16)  [unwired: 10 in]
    n161 = call "Join myDAQ DIO.vi"("IN 7"=w406, "IN 5"=w407, "IN 6, IN 4"=w408, "IN 2, IN 0"=w411, "IN 3"=w409, "IN 1"=w410) -> ("IN 7:0"=→"DIO.C_7:0.IN":u8)  [unwired: 4 in]
  }
  n162 = node-c288(w10) -> ()
